vi "testTwoServersReportConnStatus.vi"(8 "error in":errorcluster) -> (0 "error out":errorcluster)   [LabVIEW 2018]
uses:
  <vilib>/addons/_JKI Toolkits/Caraya/classes/Assert/Assert Equal Value_Variant.vi
  src/TcpServer/TcpServer.lvclass
  <vilib>/addons/_JKI Toolkits/Caraya/classes/Test/Test.lvclass
  <vilib>/addons/_JKI Toolkits/Caraya/classes/Assert/Assert.lvclass
panel:
  out "Run Server B error":errorcluster
  out "Run Server A error":errorcluster
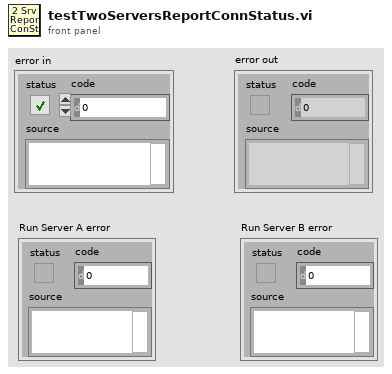
[diagram p1: front panel]
types:
  T1 = cluster{"CmdRead":refnum<user-event>, "EvtRead":refnum<user-event>, "GenRead":refnum<user-event>}
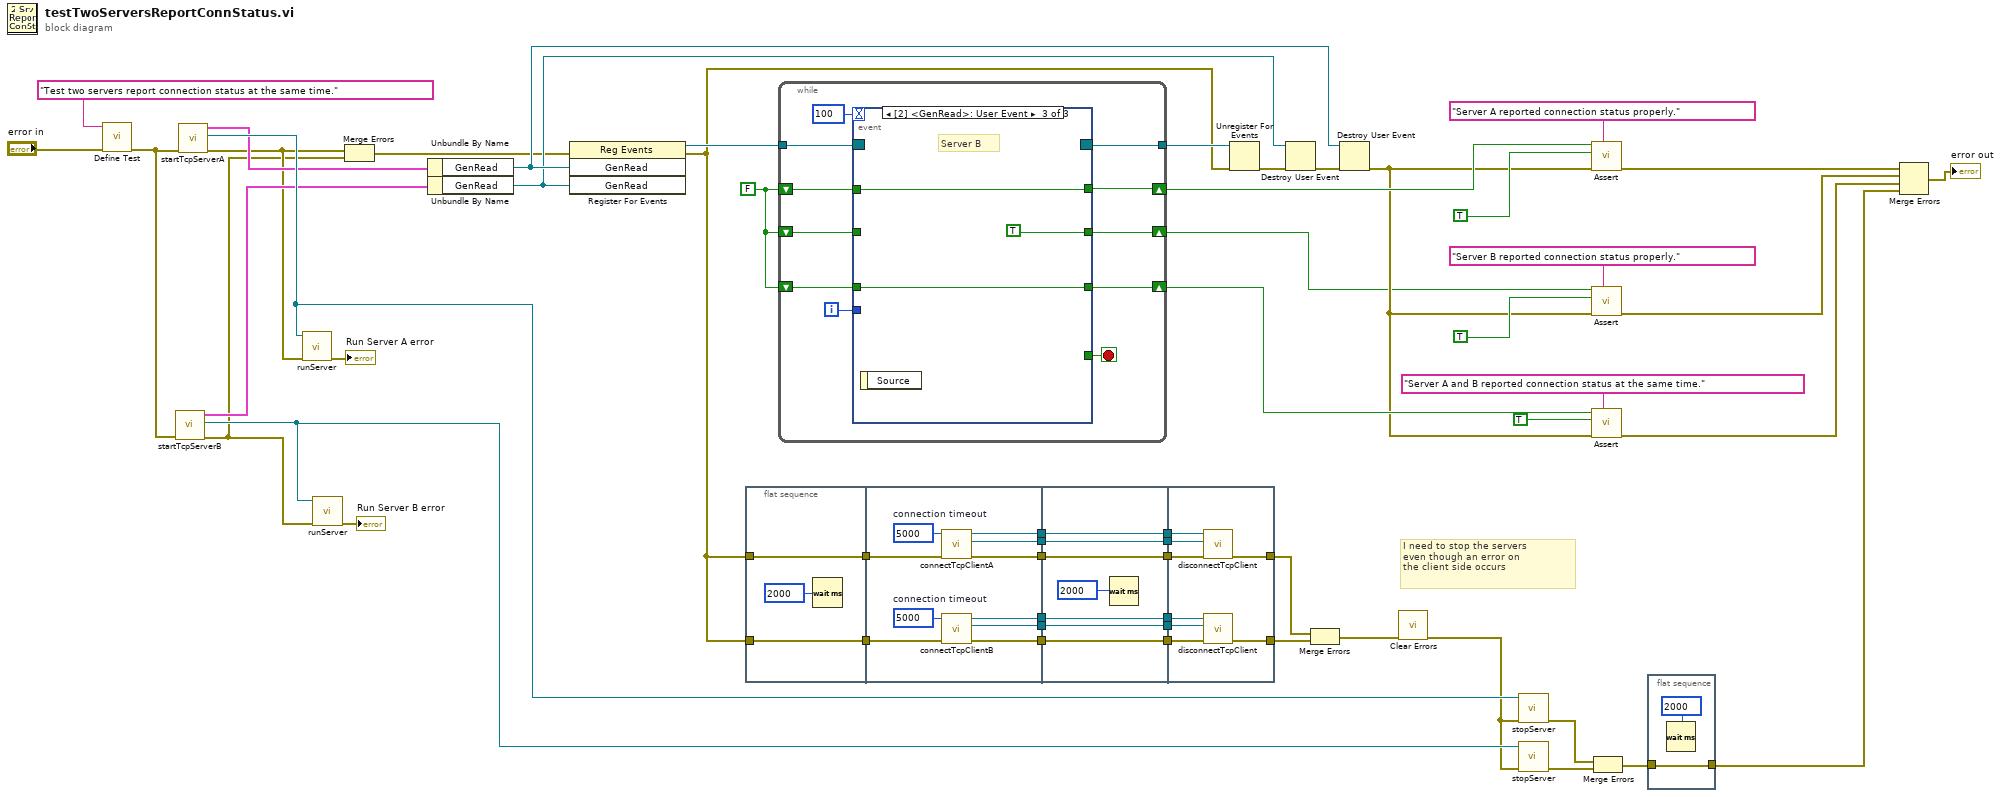
[diagram p0: block diagram]
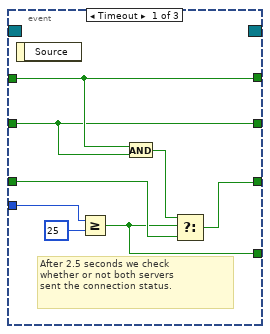
[diagram p2: hidden frame]
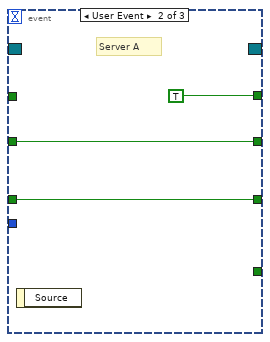
[diagram p3: hidden frame]
diagram:
  w1 = FALSE ("connStatus")
  # "I need to stop the servers \neven though an error on \nthe client side occurs"
  n1 = call <vilib>:"Define Test.vi"("error in (no error)"="error in", "Label (VI Title)"="Test two servers report connection status at the same time.") -> ("error out"=w48:errorcluster)  [unwired: 9 in]
  n2 = call "startTcpServerB.vi"("error in (no error)"=w48) -> ("error out"=w2:errorcluster, "TcpServer out"=w53:refnum<class "TcpServer.lvclass">, "UserEvents"=w45:T1)  [unwired: 8 in]
  n3 = call "startTcpServerA.vi"("error in (no error)"=w48) -> ("error out"=w23:errorcluster, "TcpServer out"=w47:refnum<class "TcpServer.lvclass">, "UserEvents"=w46:T1)  [unwired: 8 in]
  n4 = call "runServer.vi"("error in (no error)"=w23, "TcpServer in"=w47) -> ("error out (no error)"=→"Run Server A error":errorcluster)  [unwired: 8 in, 1 out]
  n5 = call "runServer.vi"("error in (no error)"=w2, "TcpServer in"=w53) -> ("error out (no error)"=→"Run Server B error":errorcluster)  [unwired: 8 in, 1 out]
  n6 = Merge Errors(w23, w2) -> (w3:errorcluster)
  n7 = Unbundle By Name(w46) -> ("GenRead"=w26:refnum<user-event>)
  n8 = Unbundle By Name(w45) -> ("GenRead"=w18:refnum<user-event>)
  n9 = register-events(error in=w3, w26, w18) -> (reference out=w44:refnum<event-registration>, error out=w4:errorcluster)  [unwired: 1 in]
  n10 = flat-sequence {
    tunnel: [w58] -> w6
    tunnel: w4 -> [w58]
    tunnel: [w57] -> w5
    tunnel: w4 -> [w57]
    tunnel: [w69] -> w42
    tunnel: [w68] -> w40
    tunnel: [w67] -> w38
    tunnel: [w66] -> w36
    tunnel: [w65] -> w34
    tunnel: [w64] -> w32
    tunnel: w6 -> [w63]
    tunnel: w5 -> [w62]
    tunnel: [w75] -> w43
    tunnel: w42 -> [w75]
    tunnel: [w74] -> w41
    tunnel: w40 -> [w74]
    tunnel: [w73] -> w39
    tunnel: w38 -> [w73]
    tunnel: [w72] -> w37
    tunnel: w36 -> [w72]
    tunnel: [w71] -> w35
    tunnel: w34 -> [w71]
    tunnel: [w70] -> w33
    tunnel: w32 -> [w70]
    tunnel: w43 -> [w84]
    tunnel: w41 -> [w83]
    tunnel: w39 -> [w82]
    tunnel: w37 -> [w81]
    tunnel: w35 -> [w80]
    tunnel: w33 -> [w79]
    tunnel: [w78] -> w30
    tunnel: [w77] -> w29
    frame #0 {
      n11 = Wait (ms)(milliseconds to wait=u32 2000) -> ()  [unwired: 1 out]
    }
    frame #1 {
      w60 = 5000  # connection timeout
      w61 = 5000  # connection timeout
      n12 = call "connectTcpClientA.vi"("error in (no error)"=w63, "connection timeout (ms)"=w61) -> ("error out"=w67:errorcluster, "tel connection ID A out"=w68:refnum<k5>, "cmd connection ID A out"=w69:refnum<k5>)  [unwired: 7 in]
      n13 = call "connectTcpClientB.vi"("error in (no error)"=w62, "connection timeout (ms)"=w60) -> ("error out"=w64:errorcluster, "tel connection ID B out"=w65:refnum<k5>, "cmd connection ID B out"=w66:refnum<k5>)  [unwired: 7 in]
    }
    frame #2 {
      n14 = Wait (ms)(milliseconds to wait=u32 2000) -> ()  [unwired: 1 out]
    }
    frame #3 {
      n15 = call "disconnectTcpClient.vi"("error in (no error)"=w82, "tel connection ID in"=w83, "cmd connection ID in"=w84) -> ("error out"=w78:errorcluster)  [unwired: 8 in]
      n16 = call "disconnectTcpClient.vi"("error in (no error)"=w79, "tel connection ID in"=w80, "cmd connection ID in"=w81) -> ("error out"=w77:errorcluster)  [unwired: 8 in]
    }
  }
  n17 = while {
    tunnel: [w95] -> w31
    tunnel: w44 -> [w93]
    shift-right: [w92] -> w17
    shift-left: w1 -> [w91]
    shift-right: [w89] -> w7
    shift-left: w1 -> [w90]
    shift-right: [w88] -> w12
    shift-left: w1 -> [w87]
    i -> [w86]
    stop <- w85 stop-if-true
    # "Event Structure for TCP server A"
    n18 = event shown="[2] <GenRead>: User Event" {
      selector: w93 -> [_ _ _]
      dyn-events: [_ _ _] -> w95
      timeout: 100 -> [_ _ _]
      tunnel: [w97 TRUE w109] -> w92
      tunnel: w91 -> [w97 _ w109]
      tunnel: [w96 w104 TRUE] -> w89
      tunnel: w90 -> [w96 w104 _]
      tunnel: [w99 w106 w108] -> w88
      tunnel: w87 -> [w101 w106 w108]
      tunnel: w86 -> [w102 _ _]
      tunnel: [w98 _ _] -> w85
      event Timeout {
        # "After 2.5 seconds we check\nwhether or not both servers\nsent the connection status."
        n19 = event-data() -> ()  [unwired: 1 in, 1 out]
        n20 = Greater Or Equal?(x=w102, y=25) -> (x >= y?=w98:bool)
        n21 = And(x=w97, y=w96) -> (x .and. y?=w100:bool)
        n22 = Select(t=w100, s=w98, f=w101) -> (s? t:f=w99:bool)
      }
      event User Event {
        # "Server A"
        n23 = event-data() -> ()  [unwired: 1 in, 1 out]
      }
      event User Event {
        # "Server B"
        n24 = event-data() -> ()  [unwired: 1 in, 1 out]
      }
    }
  }
  n25 = Unregister For Events(event registration refnum=w31, error in=w4) -> (error out=w20:errorcluster)
  n26 = Destroy User Event(user event=w18, error in=w20) -> (error out=w19:errorcluster)
  n27 = Merge Errors(w30, w29) -> (w28:errorcluster)
  n28 = Destroy User Event(user event=w26, error in=w19) -> (error out=w11:errorcluster)
  n29 = call <vilib>:"Clear Errors.vi"("error in (no error)"=w28) -> ("error out"=w27:errorcluster)  [unwired: 5 in, 1 out]
  n30 = call "stopServer.vi"("error in (no error)"=w27, "tcpServer in"=w47) -> ("error out"=w52:errorcluster)  [unwired: 8 in, 1 out]
  n31 = call "stopServer.vi"("error in (no error)"=w27, "tcpServer in"=w53) -> ("error out"=w51:errorcluster)  [unwired: 8 in, 1 out]
  n32 = call-poly <vilib>:"Assert.vi"("Label"="Server A reported connection status properly.", "error in (no error)"=w11, "Y"=TRUE ("Boolean"), "X"=w17) -> ("error out"=w21:errorcluster)  [unwired: 7 in]
  n33 = call-poly <vilib>:"Assert.vi"("Label"="Server B reported connection status properly.", "error in (no error)"=w11, "Y"=TRUE ("Boolean"), "X"=w7) -> ("error out"=w9:errorcluster)  [unwired: 7 in]
  n34 = call-poly <vilib>:"Assert.vi"("Label"="Server A and B reported connection status at the same time.", "error in (no error)"=w11, "Y"=TRUE ("connStatus"), "X"=w12) -> ("error out"=w8:errorcluster)  [unwired: 7 in]
  n35 = Merge Errors(w52, w51) -> (w50:errorcluster)
  n36 = flat-sequence {
    tunnel: w50 -> [w110]
    tunnel: [w110] -> w10
    frame #0 {
      n37 = Wait (ms)(milliseconds to wait=u32 2000) -> ()  [unwired: 1 out]
    }
  }
  n38 = Merge Errors(w21, w9, w8, w10) -> (→"error out":errorcluster)
